vi "Wait for Time.vi"() -> ()   [LabVIEW 2014]
panel:
  in  "Time Stamp":timestamp format="%<%X\n%x>T"
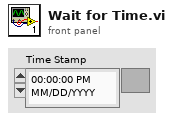
[diagram p1: front panel]
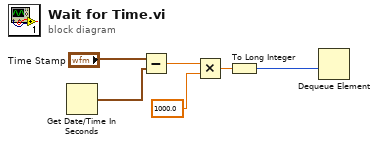
[diagram p0: block diagram]
diagram:
  n1 = Get Date/Time In Seconds() -> (seconds since 1Jan1904=w5:timestamp)
  n2 = Subtract(x="Time Stamp", y=w5) -> (x-y=w4:dbl)
  n3 = Multiply(x=w4, y=1000.0) -> (x*y=w2:dbl)
  n4 = To Long Integer(number=w2) -> (32bit integer=w1:i32)
  n5 = Dequeue Element(timeout in ms (-1)=w1) -> ()  [unwired: 2 in, 4 out]
